vi "Page_Source_Can_Add_to_Top.vi"(6 "Project Refnum":refnum<vi>, 8 "error in (no error)":errorcluster, 10 "AB_Source in":refnum<class "AB_Source.lvclass">, 11 "AB_WebService in":refnum<class "AB_WebService.lvclass">) -> (0 "error out":errorcluster, 1 "message":string, 2 "canAddToTop":bool, 3 "AB_WebService out":refnum<class "AB_WebService.lvclass">)   [LabVIEW 2020, in "AB_WebService.lvclass"]
uses:
  <vilib>/AppBuilder/AB_Classes/WebService/AB_WebService.lvclass
  <vilib>/AppBuilder/AB_Classes/Source/AB_Source.lvclass
  <resource>/Framework/Providers/Common/provcom_StringGlobals.vi
  <vilib>/AppBuilder/AB_Classes/TargetFile/AB_Targetfile.lvclass
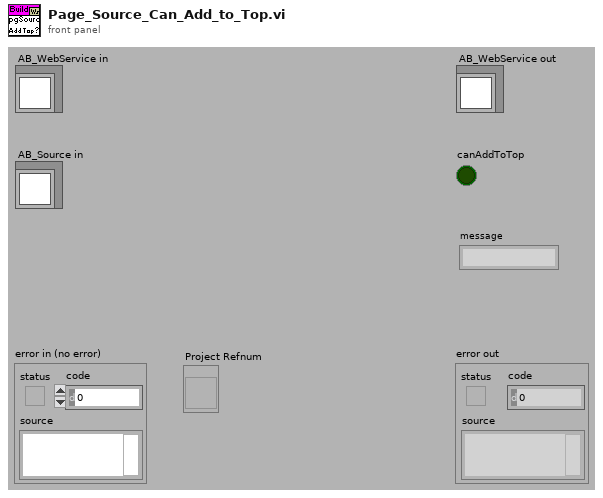
[diagram p1: front panel]
types:
  T1 = typedef "AB_Source.ctl" = cluster{"path":path, "itemID":string, "parentIndex":i32, "sourceInclusion":T2, "destinationIndex":i32, "properties":T3[], "newName":string, "lvfile":bool, "valid":bool, "eng_inBuild":bool, "eng_isNonVILink":bool, "Amalgamation":bool, "Amalgamation Piece":bool, "eng_delimitedName":string, "preventRename":bool}
  T2 = typedef "AB_Source_Inclusion.ctl" = enum16{"IncludeIfReferenced", "Include", "Exclude", "TopLevel"}
  T3 = typedef "AB_Source_Properties.ctl" = cluster{"sourcePropertyType":T4, "value":variant}
  T4 = typedef "AB_Source_Property_Type.ctl" = enum16{"Remove block diagram", "Remove front panel", "Password", "Window has title bar", "Show menu bar", "Show vertical scroll bar", "Show horizontal scroll bar", "Show toolbar", "Show Abort button", "Show fp when called", "Window behavior", "Allow user to close window", "Window run-time position", "Run when opened", "Allow debugging", "Auto error handling", "Generate guard code", "Use stack variables", "Expression folding", "Integer only", "Inline subVI"}
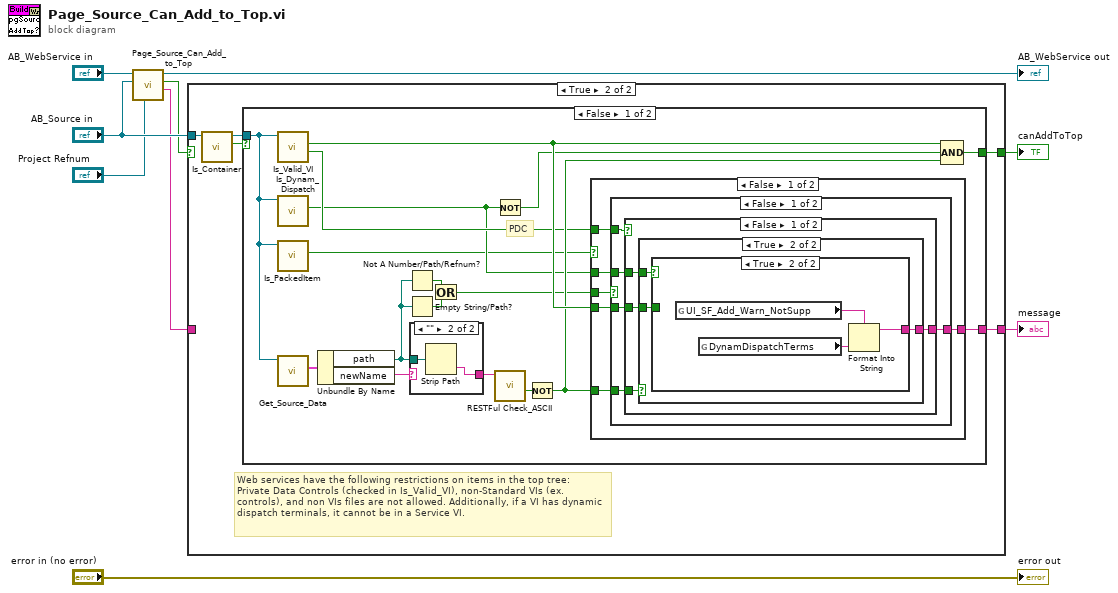
[diagram p0: block diagram]
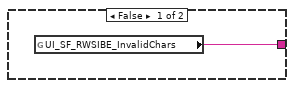
[diagram p3: hidden frame]
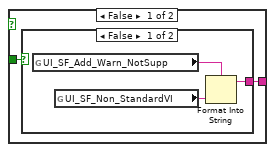
[diagram p4: hidden frame]
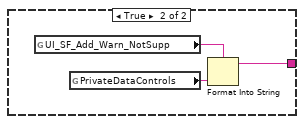
[diagram p6: hidden frame]
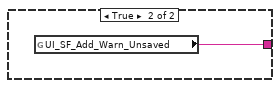
[diagram p7: hidden frame]
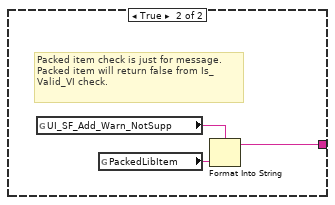
[diagram p8: hidden frame]
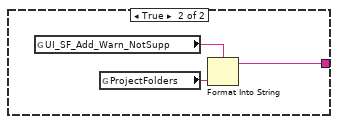
[diagram p10: hidden frame]
diagram:
  n1 = call-parent "Page_Source_Can_Add_to_Top.vi"("Project Refnum"="Project Refnum", "AB_Source in"="AB_Source in", "AB_Targetfile in"="AB_WebService in") -> ("message"=w2:string, "canAddToTop"=w3:bool, "AB_Targetfile out"=→"AB_WebService out":refnum<class "AB_WebService.lvclass">)  [unwired: 5 in, 1 out]
  n2 = case shown="True" w3 {
    selector: w3 -> [w10 _]
    tunnel: [w10 w14] -> w8
    tunnel: [w11 w13] -> w7
    tunnel: "AB_Source in" -> [_ w12]
    tunnel: w2 -> [w11 _]
    frame False {
    }
    frame True {
      # "Web services have the following restrictions on items in the top tree:\nPrivate Data Controls (checked in Is_Valid_VI), non-Standard VIs (ex. controls), and non VIs files are not allowed. Additionally, if a VI has dynamic dispatch terminals, it cannot be in a Service VI."
      n3 = call-dynamic "Is_Container.vi"("AB_Source in"=w12) -> ("container"=w16:bool, "AB_Source out"=w15:refnum<class "AB_Source.lvclass">)  [unwired: 8 in, 1 out]
      n4 = case shown="False" w16 {
        tunnel: w15 -> [w18 _]
        tunnel: [w33 _] -> w14
        tunnel: [w20 w71] -> w13
        frame False {
          # "PDC"
          n5 = call-dynamic "Is_Valid_VI.vi"("AB_Source in"=w18) -> ("PDC"=w22:bool, "VI"=w25:bool)  [unwired: 7 in, 2 out]
          n6 = call-dynamic "Is_Dynam_Dispatch.vi"("AB_Source in"=w18) -> ("dynamicDispatch"=w19:bool)  [unwired: 8 in, 2 out]
          n7 = call-dynamic "Is_PackedItem.vi"("AB_Source in"=w18) -> ("packed item"=w17:bool)  [unwired: 8 in, 2 out]
          n8 = call <vilib>:"Get_Source_Data.vi"("Class in"=w18) -> ("data"=w32:T1)  [unwired: 8 in, 2 out]
          n9 = Unbundle By Name(w32) -> ("path"=w28:path, "newName"=w31:string)
          n10 = Not A Number/Path/Refnum?(number/path/refnum=w28) -> (NaN/Path/Refnum?=w27:bool)
          n11 = Empty String/Path?(string/path=w28) -> (empty?=w26:bool)
          n12 = case shown="\"\"" w31 {
            selector: w31 -> [w68 _]
            tunnel: w28 -> [_ w70]
            tunnel: [w68 w69] -> w30
            frame Default {
            }
            frame "" {
              n13 = Strip Path(path=w70) -> (name=w69:string)  [unwired: 1 out]
            }
          }
          n14 = Or(x=w27, y=w26) -> (x .or. y?=w21:bool)
          n15 = Not(x=w19) -> (.not. x?=w24:bool)
          n16 = call <vilib>:"RESTFul Check_ASCII.vi"("string in"=w30) -> ("invalid chars?"=w29:bool)  [unwired: 9 in, 1 out]
          n17 = Not(x=w29) -> (.not. x?=w23:bool)
          n18 = case shown="False" w17 {
            tunnel: w25 -> [w39 _]
            tunnel: w23 -> [w38 _]
            tunnel: w22 -> [w37 _]
            tunnel: w21 -> [w36 _]
            tunnel: [w35 w65] -> w20
            tunnel: w19 -> [w34 _]
            frame False {
              n19 = case shown="False" w36 {
                tunnel: w39 -> [w40 _]
                tunnel: w34 -> [w42 _]
                tunnel: w38 -> [w41 _]
                tunnel: w37 -> [w44 _]
                tunnel: [w43 w64] -> w35
                frame False {
                  n20 = case shown="False" w44 {
                    tunnel: [w48 w61] -> w43
                    tunnel: w42 -> [w45 _]
                    tunnel: w41 -> [w47 _]
                    tunnel: w40 -> [w46 _]
                    frame False {
                      n21 = case shown="True" w47 {
                        tunnel: [w49 w51] -> w48
                        tunnel: w46 -> [_ w50]
                        tunnel: w45 -> [_ w52]
                        frame False {
                          n22 = global read "provcom_StringGlobals.vi" "UI_SF_RWSIBE_InvalidChars"() -> (w49:string)
                        }
                        frame True {
                          n23 = case shown="True" w52 {
                            tunnel: [w53 w58] -> w51
                            tunnel: w50 -> [w54 _]
                            frame False {
                              n24 = case shown="False" w54 {
                                tunnel: [w55 _] -> w53
                                frame False {
                                n25 = global read "provcom_StringGlobals.vi" "UI_SF_Add_Warn_NotSupp"() -> (w57:string)
                                n26 = global read "provcom_StringGlobals.vi" "UI_SF_Non_StandardVI"() -> (w56:string)
                                n27 = Format Into String(format string=w57, w56) -> (resulting string=w55:string)  [unwired: 2 in, 1 out]
                                }
                                frame True {
                                }
                              }
                            }
                            frame True {
                              n28 = global read "provcom_StringGlobals.vi" "UI_SF_Add_Warn_NotSupp"() -> (w60:string)
                              n29 = global read "provcom_StringGlobals.vi" "DynamDispatchTerms"() -> (w59:string)
                              n30 = Format Into String(format string=w60, w59) -> (resulting string=w58:string)  [unwired: 2 in, 1 out]
                            }
                          }
                        }
                      }
                    }
                    frame True {
                      n31 = global read "provcom_StringGlobals.vi" "UI_SF_Add_Warn_NotSupp"() -> (w63:string)
                      n32 = global read "provcom_StringGlobals.vi" "PrivateDataControls"() -> (w62:string)
                      n33 = Format Into String(format string=w63, w62) -> (resulting string=w61:string)  [unwired: 2 in, 1 out]
                    }
                  }
                }
                frame True {
                  n34 = global read "provcom_StringGlobals.vi" "UI_SF_Add_Warn_Unsaved"() -> (w64:string)
                }
              }
            }
            frame True {
              # "Packed item check is just for message. Packed item will return false from Is_Valid_VI check."
              n35 = global read "provcom_StringGlobals.vi" "UI_SF_Add_Warn_NotSupp"() -> (w67:string)
              n36 = global read "provcom_StringGlobals.vi" "PackedLibItem"() -> (w66:string)
              n37 = Format Into String(format string=w67, w66) -> (resulting string=w65:string)  [unwired: 2 in, 1 out]
            }
          }
          n38 = Compound Arithmetic op=AND(w25, w24, w23) -> (w33:bool)
        }
        frame True {
          n39 = global read "provcom_StringGlobals.vi" "UI_SF_Add_Warn_NotSupp"() -> (w73:string)
          n40 = global read "provcom_StringGlobals.vi" "ProjectFolders"() -> (w72:string)
          n41 = Format Into String(format string=w73, w72) -> (resulting string=w71:string)  [unwired: 2 in, 1 out]
        }
      }
    }
  }
  "canAddToTop" <- w8
  "message" <- w7
  "error out" <- "error in (no error)"
